vi "_Analyze Cache Size.vi"(8 "error in (no error)":errorcluster, 11 "DataSize":i32) -> (0 "error out":errorcluster, 3 "CacheSize":i32)   [LabVIEW 2017, in "MDPtr.lvlib" / "MDPtrMgr.lvclass"]
uses:
  MDPtrMgr.lvclass
  56ab45e0-4a17-45e8-867a-270e4bd861ae.vi
  MDPtr.lvlib
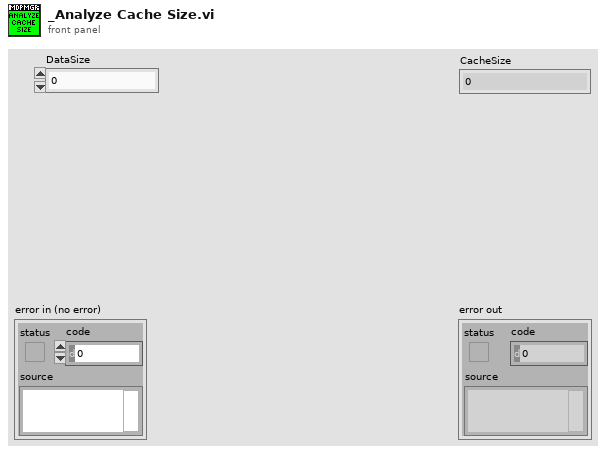
[diagram p1: front panel]
types:
  T1 = typedef "MDPtr.lvlib/Def-GlobalSettings.ctl" = cluster{"Malloc Method":T2, "FixedPreSize":cluster{"PreCacheSize":i32}}
  T2 = typedef "MDPtr.lvlib/MDPtr MallocMethod.ctl" = enum16{"NONE", "FIXED PRE-SIZE"}
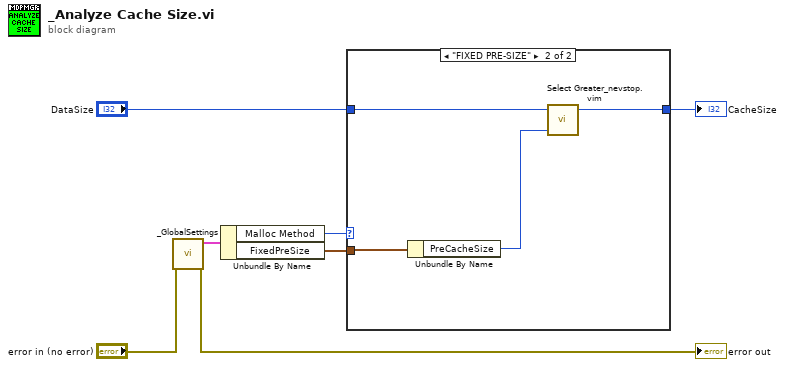
[diagram p0: block diagram]
diagram:
  n1 = call "_GlobalSettings.vi"("error in (no error)"="error in (no error)") -> ("error out"=→"error out":errorcluster, "Setting out"=w7:T1)  [unwired: 9 in]
  n2 = Unbundle By Name(w7) -> ("Malloc Method"=w6:T2, "FixedPreSize"=w1:cluster{"PreCacheSize":i32})
  n3 = case shown="\"FIXED PRE-SIZE\"" w6 {
    tunnel: [w8 w9] -> w5
    tunnel: "DataSize" -> [w8 w11]
    tunnel: w1 -> [_ w12]
    frame "NONE", Default {
    }
    frame "FIXED PRE-SIZE" {
      n4 = Unbundle By Name(w12) -> ("PreCacheSize"=w10:i32)
      n5 = call "Select Greater_nevstop.vim"("A"=w11, "B"=w10) -> ("lesser"=w9:i32)  [unwired: 3 in]
    }
  }
  "CacheSize" <- w5
